vi "Autonomous Independent.vi"() -> ()   [LabVIEW 2017]
doc: "This VI is called when autonomous begins, and will automatically be terminated when autonomous ends. You can carry out timed or sensor driven robot movement independently without needing to return to the caller."
uses:
  <vilib>/Rock Robotics/WPI/Relay/WPI_RelayValue.ctl
  <vilib>/Rock Robotics/WPI/Utilities/WPI_GetSetVariantRefNum.vi
  <vilib>/Rock Robotics/Network Tables/NT Read String.vi
  Robot Global Data.vi
  <vilib>/Rock Robotics/WPI/RobotDrive/WPI_RobotDriveArcadeDrive_Standard(NoSaturation).vi
  <vilib>/Rock Robotics/Network Tables/NT Write Numeric Array.vi
panel:
  out "Current Movement, for debugging":T1 {"Y Joystick Value" scale=1.0..-1.0; "X Joystick Value" scale=-1.0..1.0}
  in  "Array of robot movements":T2(array[cluster])=[{"X Joystick Value"=0.39393939393939403, "Y Joystick Value"=0.0, "Delay (sec)"=1.0, "Movement Name"="turn"}, {"X Joystick Value"=-0.3737373737373737, "Y Joystick Value"=0.0, "Delay (sec)"=1.0, "Movement Name"="turn back"}] {"Y Joystick Value" scale=1.0..-1.0; "X Joystick Value" scale=-1.0..1.0}
  # "Be sure to right-click and choose Data Operations>>Make Current Value default if you want to save the array values with the VI"
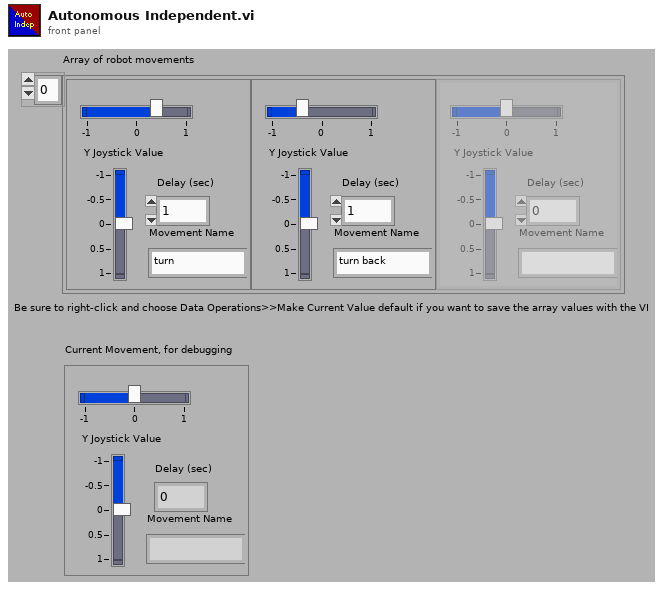
[diagram p1: front panel]
types:
  T1 = cluster{"X Joystick Value":dbl, "Y Joystick Value":dbl, "Delay (sec)":dbl, "Movement Name":string}
  T2 = cluster{"X Joystick Value":dbl, "Y Joystick Value":dbl, "Delay (sec)":dbl, "Movement Name":string}[]
  T3 = typedef "WPI_JoystickDevRef.ctl" = cluster{"Device":T4}
  T4 = typedef "WPI_JoystickDeviceEnum.ctl" = enum16{"USB 0", "USB 1", "USB 2", "USB 3", "USB 4", "USB 5"}
  T5 = typedef "WPI_RelayValue.ctl" = enum16{"Off", "On", "Forward", "Reverse"}
  T6 = cluster{"Distance (ft)":dbl, "Score":dbl, "Normalized":cluster{"Center":cluster{dbl, dbl}, "Rectangle":cluster{"Numeric":dbl, "Numeric 2":dbl, "Numeric 3":dbl, "Numeric 5":dbl}}, "Pixels":cluster{"Center":cluster{dbl, dbl}, "Rectangle":cluster{"Numeric":dbl, "Numeric 2":dbl, "Numeric 3":dbl, "Numeric 5":dbl}}}
  T7 = typedef "WPI_RelayDevRef.ctl" = cluster{"DevStatus":errorcluster, "Relay Channel":T8, "Relay Direction":T9}
  T8 = typedef "FPGA_DIORelayChannel.ctl" = enum8{"Relay 0", "Relay 1", "Relay 2", "Relay 3", "Invalid"}
  T9 = typedef "WPI_RelayDirection.ctl" = enum16{"Both directions", "Forward only", "Reverse only"}
  T10 = typedef "WPI_RobotDriveDevRef.ctl" = cluster{"DevStatus":errorcluster, "Motors[]":T11[], "Square Inputs":bool, "Max Output":dbl}
  T11 = typedef "WPI_MotorControlDeviceRef.ctl" = cluster{"DeviceStatus":errorcluster, "Type":T12, "PWM":cluster{"PWM Channel":T13, "DeadBand":T14}, "CAN":cluster{"Device Number":u8, "SetOutput VI Ref":variant, "GetOutput VI Ref":variant, "Enable VI Ref":variant, "Disable VI Ref":variant, "Data":variant}, "Invert":bool, "DIO PWM":cluster{"PWM \"Enable\" Channel":T13, "DIOChannel":T15, "PWM Rate":dbl}}
  T12 = typedef "WPI_MotorControlType.ctl" = enum16{"PWM", "CAN", "DIO PWM"}
  T13 = typedef "FPGA_DIOPWMChannel.ctl" = enum8{"PWM 0", "PWM 1", "PWM 2", "PWM 3", "PWM 4", "PWM 5", "PWM 6", "PWM 7", "PWM 8", "PWM 9", "PWM MXP 0", "PWM MXP 1", "PWM MXP 2", "PWM MXP 3", "PWM MXP 4", "PWM MXP 5", "PWM MXP 6", "PWM MXP 7", "PWM MXP 8", "PWM MXP 9", "Invalid"}
  T14 = typedef "WPI_PWMDeadband.ctl" = cluster{"Name":string, "maxPositivePwm":i32, "minPositivePwm":i32, "centerPwm":i32, "maxNegativePwm":i32, "minNegativePwm":i32, "angularRange":u16}
  T15 = typedef "FPGA_DIOChannel.ctl" = enum8{"DIO 0", "DIO 1", "DIO 2", "DIO 3", "DIO 4", "DIO 5", "DIO 6", "DIO 7", "DIO 8", "DIO 9", "DIO MXP 0", "DIO MXP 1", "DIO MXP 2", "DIO MXP 3", "DIO MXP 4", "DIO MXP 5", "DIO MXP 6", "DIO MXP 7", "DIO MXP 8", "DIO MXP 9", "DIO MXP 10", "DIO MXP 11", "DIO MXP 12", "DIO MXP 13", "DIO MXP 14", "DIO MXP 15", "SPI Port CS1", "SPI Port CS2", "SPI Port CS3", "SPI Port MISO", "SPI Port MOSI", "Invalid"}
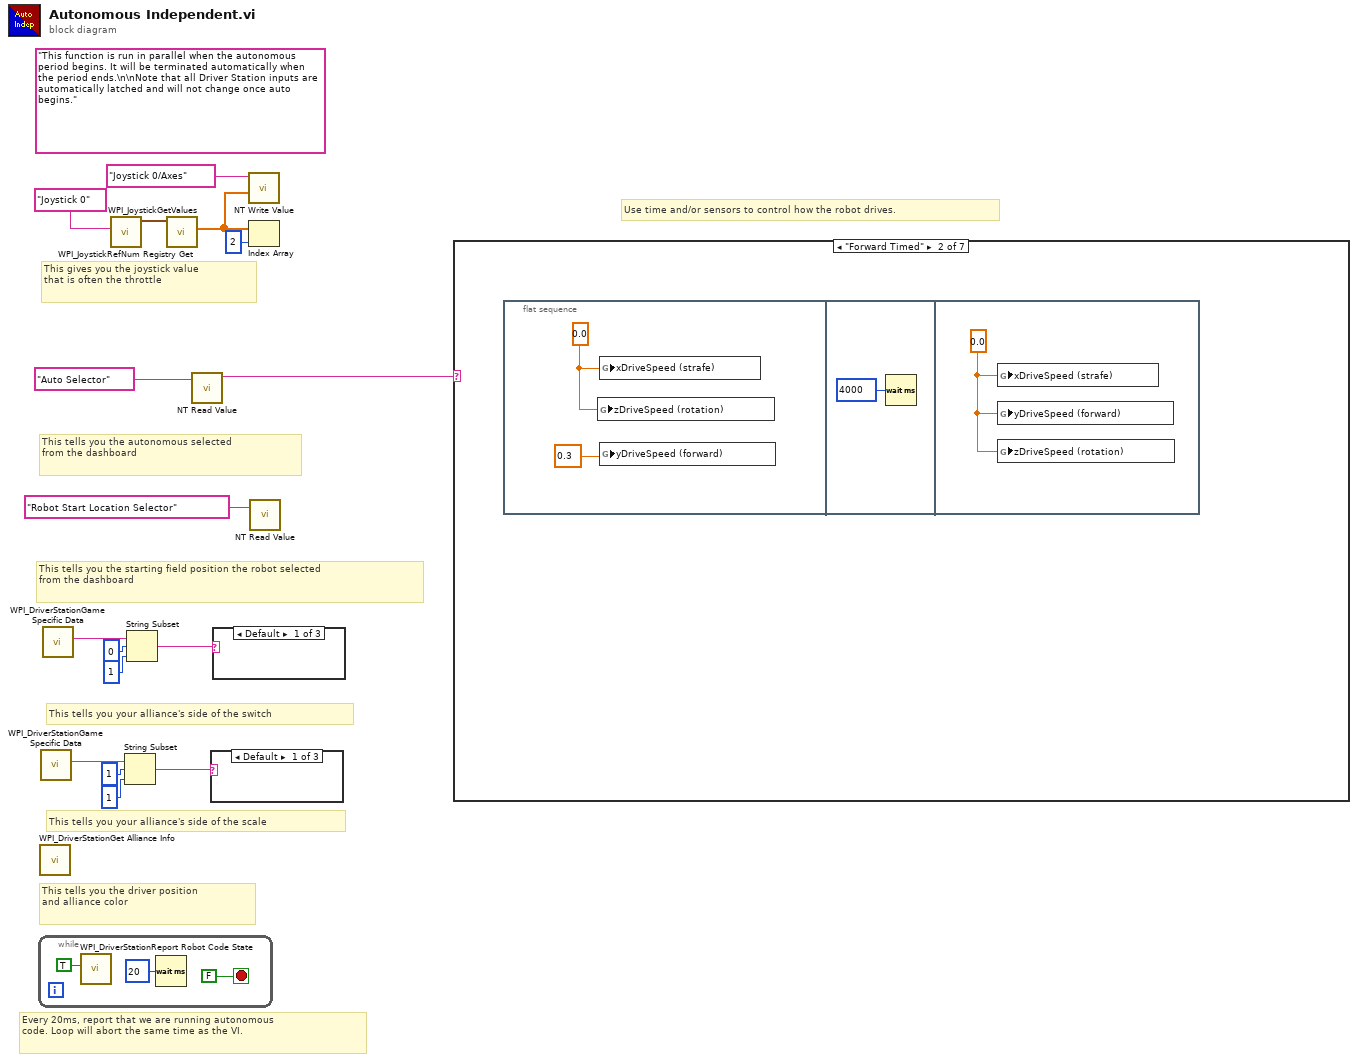
[diagram p0: block diagram]
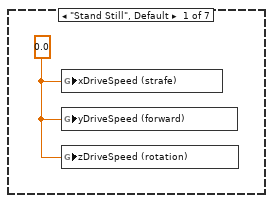
[diagram p6: hidden frame]
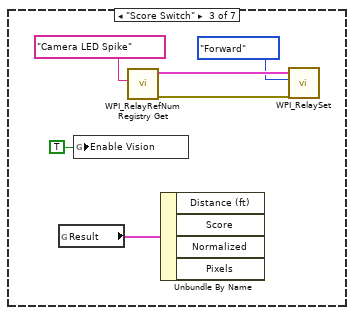
[diagram p7: hidden frame]
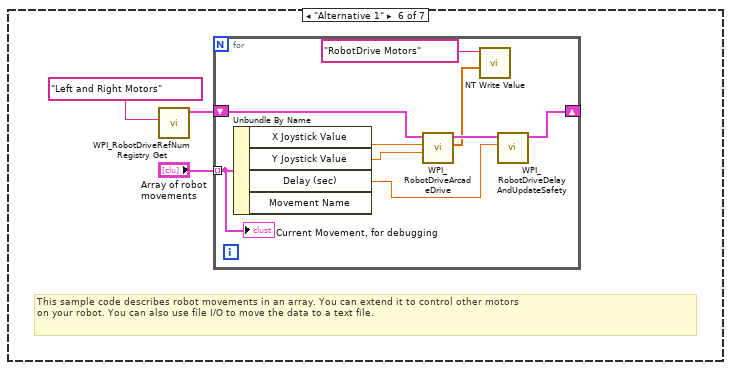
[diagram p10: hidden frame]
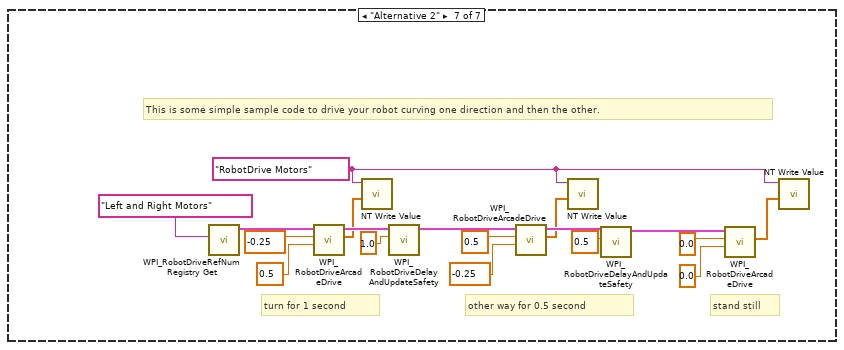
[diagram p11: hidden frame]
diagram:
  (unwired) "This function is run in parallel when the autonomous period begins. It will be terminated automatically when the period ends.\n\nNote that all Driver Station inputs are automatically latched and will not change once auto begins."
  # "This tells you your alliance's side of the scale"
  # "This tells you your alliance's side of the switch"
  # "This tells you the starting field position the robot selected\nfrom the dashboard"
  # "This tells you the autonomous selected\nfrom the dashboard"
  # "Every 20ms, report that we are running autonomous\ncode. Loop will abort the same time as the VI."
  # "This gives you the joystick value\nthat is often the throttle"
  # "Use time and/or sensors to control how the robot drives."
  # "This tells you the driver position\nand alliance color"
  n1 = while {
    stop <- FALSE stop-if-true
    n2 = call <vilib>:"WPI_DriverStationReport Robot Code State.vi"("Autonomous"=TRUE) -> ()  [unwired: 10 in, 1 out]
    n3 = Wait (ms)(milliseconds to wait=u32 20) -> ()  [unwired: 1 out]
  }
  n4 = call <vilib>:"WPI_DriverStationGet Alliance Info.vi"() -> ()  [unwired: 12 out]
  n5 = call <vilib>:"WPI_DriverStationGame Specific Data.vi"() -> ("Game Specific Data"=w5:string)  [unwired: 11 in]
  n6 = call <vilib>:"WPI_DriverStationGame Specific Data.vi"() -> ("Game Specific Data"=w9:string)  [unwired: 11 in]
  n7 = call <vilib>:"WPI_JoystickRefNum Registry Get.vi"("refnum name"="Joystick 0") -> ("JoystickDevRef"=w15:T3)  [unwired: 1 in, 9 out]
  n8 = String Subset(string=w5, offset (0)=1, length (rest)=1 ("length (rest)")) -> (substring=w3:string)
  n9 = String Subset(string=w9, offset (0)=0, length (rest)=1 ("length (rest)")) -> (substring=w7:string)
  n10 = call <vilib>:"WPI_JoystickGetValues.vi"("JoystickDevRef"=w15) -> ("Axes"=w11:dbl[])  [unwired: 6 in, 4 out]
  n11 = call-poly <vilib>:"NT Read Value.vi"("Name"="Auto Selector") -> ("String"=w12:string)  [unwired: 9 in, 1 out]
  n12 = case shown="Default" w3 {
    frame Default {
    }
    frame "L" {
    }
    frame "R" {
    }
  }
  n13 = case shown="Default" w7 {
    frame Default {
    }
    frame "L" {
    }
    frame "R" {
    }
  }
  n14 = call-poly <vilib>:"NT Write Value.vi"("Numeric Array"=w11, "Name"="Joystick 0/Axes") -> ()  [unwired: 9 in, 1 out]
  n15 = Index Array(array=w11, index=2) -> ()  [unwired: 1 out]
  n16 = call-poly <vilib>:"NT Read Value.vi"("Name"="Robot Start Location Selector") -> ()  [unwired: 9 in, 2 out]
  n17 = case shown="\"Forward Timed\"" w12 {
    frame "Stand Still", Default {
      w20 = 0.0 ("xDriveSpeed (strafe)")
      n18 = global write "Robot Global Data.vi" "xDriveSpeed (strafe)"(w20) -> ()
      n19 = global write "Robot Global Data.vi" "yDriveSpeed (forward)"(w20) -> ()
      n20 = global write "Robot Global Data.vi" "zDriveSpeed (rotation)"(w20) -> ()
    }
    frame "Forward Timed" {
      n21 = flat-sequence {
        frame #0 {
          w22 = 0.0 ("xDriveSpeed (strafe)")
          n22 = global write "Robot Global Data.vi" "zDriveSpeed (rotation)"(w22) -> ()
          n23 = global write "Robot Global Data.vi" "xDriveSpeed (strafe)"(w22) -> ()
          n24 = global write "Robot Global Data.vi" "yDriveSpeed (forward)"(0.3 ("yDriveSpeed (forward)")) -> ()
        }
        frame #1 {
          n25 = Wait (ms)(milliseconds to wait=u32 4000) -> ()  [unwired: 1 out]
        }
        frame #2 {
          w24 = 0.0 ("xDriveSpeed (strafe)")
          n26 = global write "Robot Global Data.vi" "xDriveSpeed (strafe)"(w24) -> ()
          n27 = global write "Robot Global Data.vi" "yDriveSpeed (forward)"(w24) -> ()
          n28 = global write "Robot Global Data.vi" "zDriveSpeed (rotation)"(w24) -> ()
        }
      }
    }
    frame "Score Switch" {
      n29 = global read "Robot Global Data.vi" "Result"() -> (w25:T6)
      n30 = global write "Robot Global Data.vi" "Enable Vision"(TRUE ("Enable Vision")) -> ()
      n31 = call <vilib>:"WPI_RelayRefNum Registry Get.vi"("refnum name"="Camera LED Spike") -> ("error out"=w29:errorcluster, "RelayDevRef"=w28:T7)  [unwired: 9 in]
      n32 = Unbundle By Name(w25) -> ()  [unwired: 4 out]
      n33 = call <vilib>:"WPI_RelaySet.vi"("error in (no error)"=w29, "RelayValue"=WPI_RelayValue."Forward", "RelayDevRef"=w28) -> ()  [unwired: 7 in, 2 out]
    }
    frame "Score Scale" {
    }
    frame "Deliver to Exchange" {
    }
    frame "Alternative 1" {
      # "This sample code describes robot movements in an array. You can extend it to control other motors\non your robot. You can also use file I/O to move the data to a text file."
      n34 = call <vilib>:"WPI_RobotDriveRefNum Registry Get.vi"("refnum name"="Left and Right Motors") -> ("RobotDriveDevRef"=w32:T10)  [unwired: 1 in, 9 out]
      n35 = for {
        shift-right: [w40] -> _
        shift-left: w32 -> [w41]
        tunnel: "Array of robot movements" -> [w36] mode=indexing
        n36 = Unbundle By Name(w36) -> ("X Joystick Value"=w39:dbl, "Y Joystick Value"=w38:dbl, "Delay (sec)"=w37:dbl)  [unwired: 1 out]
        n37 = call-poly <vilib>:"WPI_RobotDriveArcadeDrive.vi"("Y axis value"=w38, "X axis value"=w39, "RobotDriveDevRef"=w41) -> ("Motor Values"=w34:dbl[], "RobotDriveDevRef"=w42:T10)  [unwired: 1 in, 6 out]
        n38 = call-poly <vilib>:"NT Write Value.vi"("Numeric Array"=w34, "Name"="RobotDrive Motors") -> ()  [unwired: 9 in, 1 out]
        n39 = call <vilib>:"WPI_RobotDriveDelayAndUpdateSafety.vi"("Delay (s)"=w37, "RobotDriveDevRef"=w42) -> ("RobotDriveDevRef 2"=w40:T10)  [unwired: 8 in, 1 out]
        "Current Movement, for debugging" <- w36
      }
    }
    frame "Alternative 2" {
      w44 = "RobotDrive Motors" ("Name")
      # "This is some simple sample code to drive your robot curving one direction and then the other."
      # "stand still"
      # "other way for 0.5 second"
      # "turn for 1 second"
      n40 = call <vilib>:"WPI_RobotDriveRefNum Registry Get.vi"("refnum name"="Left and Right Motors") -> ("RobotDriveDevRef"=w60:T10)  [unwired: 1 in, 9 out]
      n41 = call-poly <vilib>:"WPI_RobotDriveArcadeDrive.vi"("Y axis value"=0.5 ("X axis value"), "X axis value"=-0.25, "RobotDriveDevRef"=w60) -> ("Motor Values"=w43:dbl[], "RobotDriveDevRef"=w53:T10)  [unwired: 1 in, 6 out]
      n42 = call-poly <vilib>:"NT Write Value.vi"("Numeric Array"=w43, "Name"=w44) -> ()  [unwired: 9 in, 1 out]
      n43 = call <vilib>:"WPI_RobotDriveDelayAndUpdateSafety.vi"("Delay (s)"=1.0, "RobotDriveDevRef"=w53) -> ("RobotDriveDevRef 2"=w54:T10)  [unwired: 8 in, 1 out]
      n44 = call-poly <vilib>:"WPI_RobotDriveArcadeDrive.vi"("Y axis value"=-0.25 ("X axis value"), "X axis value"=0.5, "RobotDriveDevRef"=w54) -> ("Motor Values"=w45:dbl[], "RobotDriveDevRef"=w55:T10)  [unwired: 1 in, 6 out]
      n45 = call-poly <vilib>:"NT Write Value.vi"("Numeric Array"=w45, "Name"=w44) -> ()  [unwired: 9 in, 1 out]
      n46 = call <vilib>:"WPI_RobotDriveDelayAndUpdateSafety.vi"("Delay (s)"=0.5, "RobotDriveDevRef"=w55) -> ("RobotDriveDevRef 2"=w56:T10)  [unwired: 8 in, 1 out]
      n47 = call-poly <vilib>:"WPI_RobotDriveArcadeDrive.vi"("Y axis value"=0.0 ("X axis value"), "X axis value"=0.0, "RobotDriveDevRef"=w56) -> ("Motor Values"=w46:dbl[])  [unwired: 1 in, 7 out]
      n48 = call-poly <vilib>:"NT Write Value.vi"("Numeric Array"=w46, "Name"=w44) -> ()  [unwired: 9 in, 1 out]
    }
  }
